vi "Set SPI CS Pin.vi"(4 "CS Active Low (T)":bool=TRUE, 5 "CS GPIO":i32=5, 8 "error in (no error)":errorcluster, 10 "CS Active":bool, 11 "VISA resource name in":refnum<visa-resource-name>) -> (0 "error out":errorcluster, 3 "VISA resource name":refnum<visa-resource-name>)   [LabVIEW 2024, in "CTIPicoVISA.lvlib"]
uses:
  CTIPicoVISA.lvlib
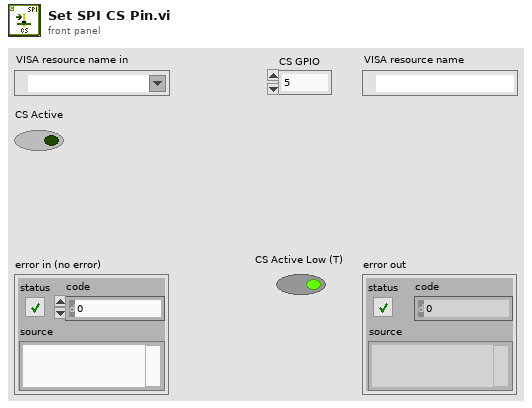
[diagram p1: front panel]
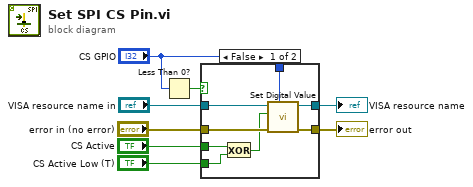
[diagram p0: block diagram]
diagram:
  n1 = Less Than 0?(x="CS GPIO") -> (x < 0?=w3:bool)
  n2 = case shown="False" w3 {
    tunnel: "error in (no error)" -> [w16 w17]
    tunnel: [w15 w17] -> w5
    tunnel: [w14 w18] -> w6
    tunnel: "VISA resource name in" -> [w13 w18]
    tunnel: "CS GPIO" -> [w11 _]
    tunnel: "CS Active" -> [w10 _]
    tunnel: "CS Active Low (T)" -> [w9 _]
    frame False {
      n3 = Exclusive Or(1:w9, 2:w10) -> (0:w12:bool)
      n4 = call "Set Digital Value.vi"("GPIO"=w11, "error in (no error)"=w16, "Value"=w12, "VISA resource name in"=w13) -> ("error out"=w15:errorcluster, "VISA resource name"=w14:refnum<visa-resource-name>)  [unwired: 6 in]
    }
    frame True {
    }
  }
  "VISA resource name" <- w6
  "error out" <- w5
